vi "calc_obj_dist.vi"(0 "Common classes":dbl[](array[numeric]), 1 "Class names":string[](array[string]), 2 "Common bboxes":dbl[][](array[numeric]), 3 "K constant":i32, 4 "X Resolution":i32) -> (5 "Object distances":cluster{string, dbl}[](array[cluster]))   [LabVIEW 2019]
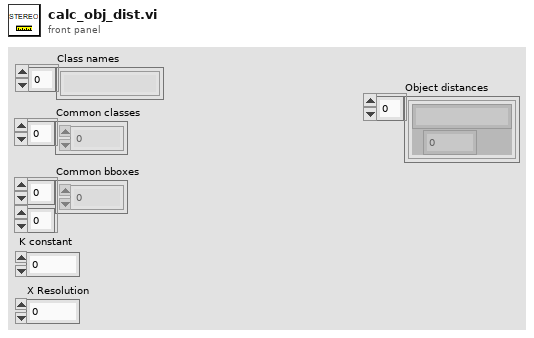
[diagram p1: front panel]
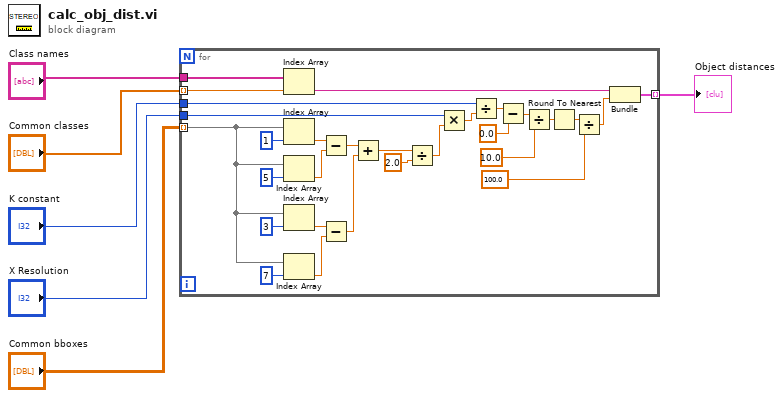
[diagram p0: block diagram]
diagram:
  n1 = for {
    tunnel: "Common bboxes" -> [w15] mode=indexing
    tunnel: "Common classes" -> [w22] mode=indexing
    tunnel: "Class names" -> [w23]
    tunnel: [w20] -> w5 mode=indexing
    tunnel: "X Resolution" -> [w18]
    tunnel: "K constant" -> [w16]
    n2 = Index Array(array=w23, index=w22) -> (element=w21:string)
    n3 = Index Array(array=w15, index=1) -> (element=w31:dbl)
    n4 = Index Array(array=w15, index=5) -> (element=w30:dbl)
    n5 = Index Array(array=w15, index=3) -> (element=w29:dbl)
    n6 = Index Array(array=w15, index=7) -> (element=w28:dbl)
    n7 = Subtract(x=w31, y=w30) -> (x-y=w27:dbl)
    n8 = Subtract(x=w29, y=w28) -> (x-y=w26:dbl)
    n9 = Add(x=w27, y=w26) -> (x+y=w25:dbl)
    n10 = Divide(x=w25, y=2.0) -> (x/y=w19:dbl)
    n11 = Multiply(x=w18, y=w19) -> (x*y=w17:dbl)
    n12 = Divide(x=w16, y=w17) -> (x/y=w14:dbl)
    n13 = Subtract(x=w14, y=0.0) -> (x-y=w12:dbl)
    n14 = Divide(x=w12, y=10.0) -> (x/y=w10:dbl)
    n15 = Round To Nearest(number=w10) -> (nearest integer value=w9:dbl)
    n16 = Divide(x=w9, y=100.0) -> (x/y=w7:dbl)
    n17 = Bundle(w21, w7) -> (w20:cluster{string, dbl})  [unwired: 1 in]
  }
  "Object distances" <- w5
